vi "BoxNetworking.vi"(8 "error in (no error)":errorcluster) -> (0 "error out":errorcluster)   [LabVIEW 2023]
uses:
  BoxNetworkingGlobal.vi
  <vilib>/Rock Robotics/Network Tables/NT Write Boolean.vi
  <vilib>/Rock Robotics/Network Tables/NT Write String.vi
  <vilib>/Rock Robotics/Network Tables/NT Write Number.vi
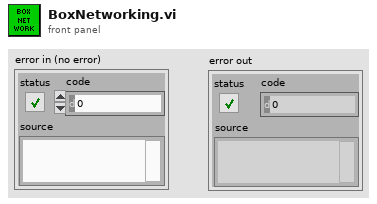
[diagram p1: front panel]
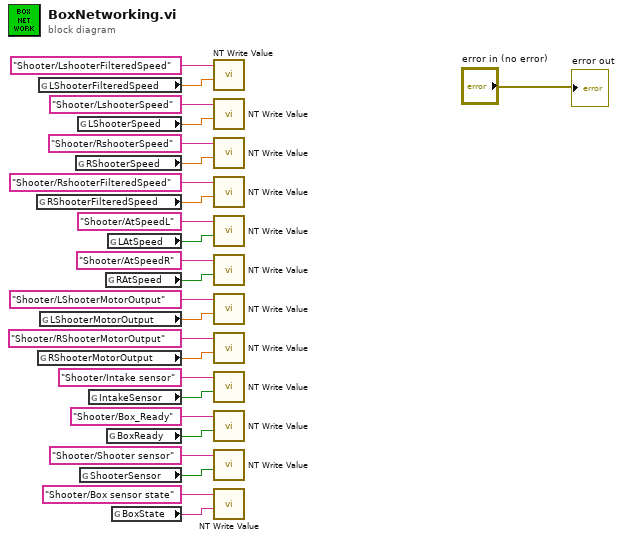
[diagram p0: block diagram]
diagram:
  n1 = global read "BoxNetworkingGlobal.vi" "RShooterFilteredSpeed"() -> (w10:dbl)
  n2 = global read "BoxNetworkingGlobal.vi" "RShooterMotorOutput"() -> (w2:dbl)
  n3 = global read "BoxNetworkingGlobal.vi" "LShooterFilteredSpeed"() -> (w16:dbl)
  n4 = global read "BoxNetworkingGlobal.vi" "LShooterMotorOutput"() -> (w4:dbl)
  n5 = global read "BoxNetworkingGlobal.vi" "RShooterSpeed"() -> (w12:dbl)
  n6 = global read "BoxNetworkingGlobal.vi" "LShooterSpeed"() -> (w14:dbl)
  n7 = global read "BoxNetworkingGlobal.vi" "ShooterSensor"() -> (w22:bool)
  n8 = global read "BoxNetworkingGlobal.vi" "IntakeSensor"() -> (w18:bool)
  n9 = global read "BoxNetworkingGlobal.vi" "RAtSpeed"() -> (w6:bool)
  n10 = global read "BoxNetworkingGlobal.vi" "BoxReady"() -> (w20:bool)
  n11 = global read "BoxNetworkingGlobal.vi" "LAtSpeed"() -> (w8:bool)
  n12 = global read "BoxNetworkingGlobal.vi" "BoxState"() -> (w25:string)
  n13 = call-poly <vilib>:"NT Write Value.vi"("value"=w16, "name"="Shooter/LshooterFilteredSpeed") -> ()  [unwired: 9 in, 1 out]
  n14 = call-poly <vilib>:"NT Write Value.vi"("value"=w14, "name"="Shooter/LshooterSpeed") -> ()  [unwired: 9 in, 1 out]
  n15 = call-poly <vilib>:"NT Write Value.vi"("value"=w12, "name"="Shooter/RshooterSpeed") -> ()  [unwired: 9 in, 1 out]
  n16 = call-poly <vilib>:"NT Write Value.vi"("value"=w10, "name"="Shooter/RshooterFilteredSpeed") -> ()  [unwired: 9 in, 1 out]
  n17 = call-poly <vilib>:"NT Write Value.vi"("value"=w8, "name"="Shooter/AtSpeedL") -> ()  [unwired: 9 in, 1 out]
  n18 = call-poly <vilib>:"NT Write Value.vi"("value"=w6, "name"="Shooter/AtSpeedR") -> ()  [unwired: 9 in, 1 out]
  n19 = call-poly <vilib>:"NT Write Value.vi"("value"=w4, "name"="Shooter/LShooterMotorOutput") -> ()  [unwired: 9 in, 1 out]
  n20 = call-poly <vilib>:"NT Write Value.vi"("value"=w2, "name"="Shooter/RShooterMotorOutput") -> ()  [unwired: 9 in, 1 out]
  n21 = call-poly <vilib>:"NT Write Value.vi"("value"=w18, "name"="Shooter/Intake sensor") -> ()  [unwired: 9 in, 1 out]
  n22 = call-poly <vilib>:"NT Write Value.vi"("value"=w20, "name"="Shooter/Box_Ready") -> ()  [unwired: 9 in, 1 out]
  n23 = call-poly <vilib>:"NT Write Value.vi"("value"=w22, "name"="Shooter/Shooter sensor") -> ()  [unwired: 9 in, 1 out]
  n24 = call-poly <vilib>:"NT Write Value.vi"("value"=w25, "name"="Shooter/Box sensor state") -> ()  [unwired: 9 in, 1 out]
  "error out" <- "error in (no error)"
